vi "Inc Dec Bearing.vi"   [LabVIEW 2014]
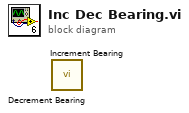
[diagram p0: block diagram]
diagram:
  n1 = call "Decrement Bearing.vi"() -> ()  [unwired: 10 in, 2 out]
  n2 = call "Increment Bearing.vi"() -> ()  [unwired: 10 in, 2 out]
